vi "Write Thing Name.vi"(8 "error in (no error)":errorcluster, 10 "Thing Name":string, 11 "Shadow Thing in":refnum<class "Thing Shadow.lvclass">) -> (0 "error out":errorcluster, 3 "Shadow Thing out":refnum<class "Thing Shadow.lvclass">)   [LabVIEW 2015, in "NI_AWS_IoT.lvlib" / "Thing Shadow.lvclass"]
uses:
  Thing Shadow.lvclass
  Thing Shadow.lvclass/Thing Shadow.ctl
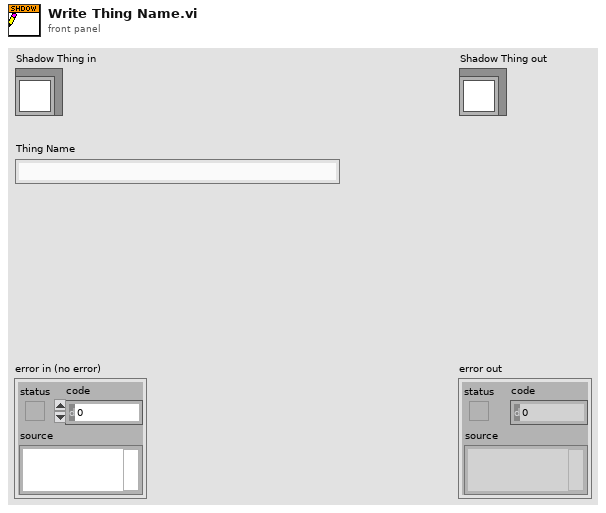
[diagram p1: front panel]
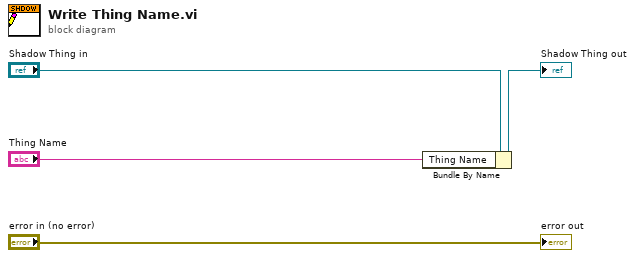
[diagram p0: block diagram]
diagram:
  n1 = Bundle By Name(cluster="Shadow Thing in", "Thing Name"="Thing Name") -> (→"Shadow Thing out":refnum<class "Thing Shadow.lvclass">)
  "error out" <- "error in (no error)"
